vi "ModStarted.vi"(10 "Caller":string, 11 "Alias":string) -> ()   [LabVIEW 2024, in "DebugTrace.lvlib"]
uses:
  DebugTrace.lvlib
  DebugTraceHandle/StartArgs.ctl
  DebugTraceHandle/DebugTraceHandle.lvclass
  DebugTraceSingleton/DebugTraceSingleton.lvlib
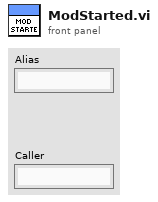
[diagram p1: front panel]
types:
  T1 = typedef "DebugTraceHandle.lvclass/StartArgs.ctl" = cluster{"Caller":string, "This":string, "Alias":string, "StartTime":timestamp}
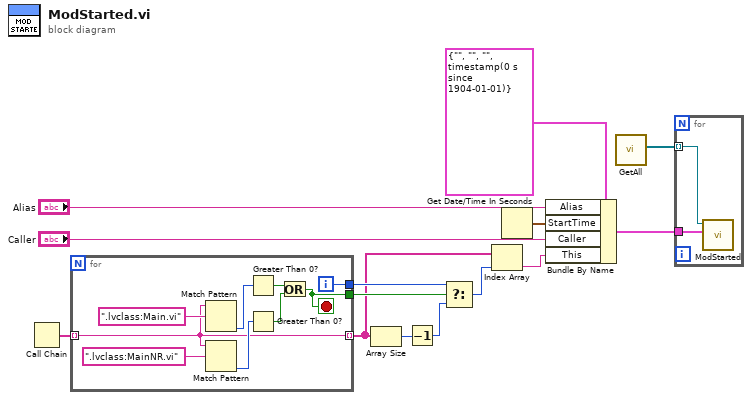
[diagram p0: block diagram]
diagram:
  n1 = Call Chain() -> (call chain=w14:string[])
  n2 = for {
    tunnel: w14 -> [w17] mode=indexing
    tunnel: [w17] -> w9 mode=indexing
    tunnel: [w16] -> w12
    tunnel: [w15] -> w13
    i -> [w16]
    stop <- w15 stop-if-true
    n3 = Match Pattern(string=w17, regular expression=".lvclass:Main.vi") -> (offset past match=w22:i32)  [unwired: 1 in, 3 out]
    n4 = Match Pattern(string=w17, regular expression=".lvclass:MainNR.vi") -> (offset past match=w21:i32)  [unwired: 1 in, 3 out]
    n5 = Greater Than 0?(x=w22) -> (x > 0?=w19:bool)
    n6 = Greater Than 0?(x=w21) -> (x > 0?=w18:bool)
    n7 = Or(x=w19, y=w18) -> (x .or. y?=w15:bool)
  }
  n8 = Array Size(array=w9) -> (size(s)=w11:i32)
  n9 = Decrement(x=w11) -> (x-1=w10:i32)
  n10 = Select(t=w12, s=w13, f=w10) -> (s? t:f=w8:i32)
  n11 = Index Array(array=w9, index=w8) -> (element=w6:string)
  n12 = Get Date/Time In Seconds() -> (seconds since 1Jan1904=w4:timestamp)
  n13 = Bundle By Name(cluster=T1 {"Caller"="", "This"="", "Alias"="", "StartTime"=timestamp(0 s since 1904-01-01)}, "Alias"="Alias", "StartTime"=w4, "Caller"="Caller", "This"=w6) -> (w1:T1)
  n14 = call "GetAll.vi"() -> ("DebugHandles"=w2:refnum<class "DebugTraceHandle.lvclass">[])  [unwired: 11 in]
  n15 = for {
    tunnel: w2 -> [w25] mode=indexing
    tunnel: w1 -> [w24]
    n16 = call-dynamic "ModStarted.vi"("StartArgs"=w24, "DebugTraceHandle"=w25) -> ()  [unwired: 10 in]
  }
